vi "receiver_framev2.vi"(8 "error in (no error)":errorcluster, 9 "Timeout(100ms)":u32=100, 11 "Visa In":refnum<visa-resource-name>) -> (0 "error out":errorcluster, 1 "TimeOut?":bool, 2 "response":string, 3 "Visa out":refnum<visa-resource-name>)   [LabVIEW 2018]
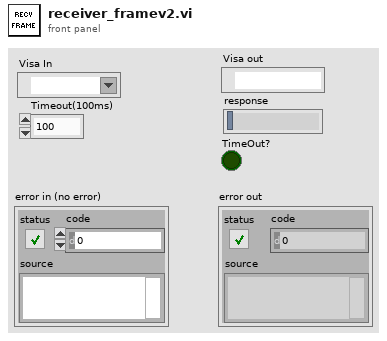
[diagram p1: front panel]
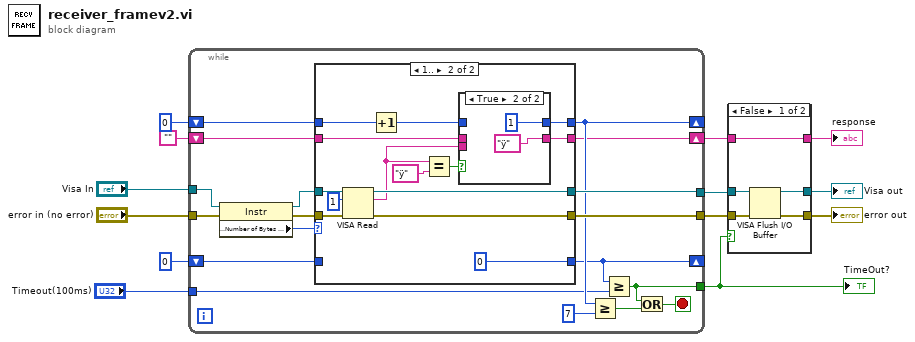
[diagram p0: block diagram]
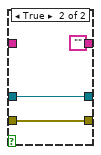
[diagram p2: hidden frame]
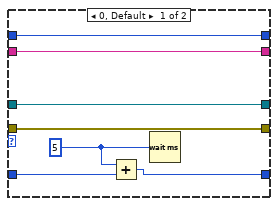
[diagram p3: hidden frame]
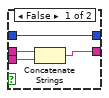
[diagram p4: hidden frame]
diagram:
  n1 = while {
    tunnel: "Visa In" -> [w31]
    tunnel: "error in (no error)" -> [w30]
    tunnel: [w26] -> w3
    tunnel: [w25] -> w7
    shift-right: [w23] -> _
    shift-left: u8 0 -> [w24]
    shift-right: [w21] -> w4
    shift-left: "" -> [w20]
    shift-right: [w14] -> _
    shift-left: u32 0 -> [w19]
    tunnel: "Timeout(100ms)" -> [w18]
    tunnel: [w15] -> w1
    stop <- w16 stop-if-true
    n2 = property class="Instr"(reference=w31, error in=w30) -> (reference out=w27:refnum<visa-resource-name>, error out=w28:errorcluster, "Serial Settings:Number of Bytes at Serial Port"=w29:u32)
    n3 = case shown="1.." w29 {
      tunnel: w28 -> [w37 w52]
      tunnel: w27 -> [w36 w51]
      tunnel: [w37 w49] -> w26
      tunnel: [w36 w48] -> w25
      tunnel: w24 -> [w38 w45]
      tunnel: [w38 w46] -> w23
      tunnel: [w35 w43] -> w21
      tunnel: w20 -> [w35 w42]
      tunnel: w19 -> [w32 _]
      tunnel: [w33 u32 0] -> w14
      frame 0, Default {
        w34 = u32 5 ("milliseconds to wait")
        n4 = Add(x=w34, y=w32) -> (x+y=w33:u32)
        n5 = Wait (ms)(milliseconds to wait=w34) -> ()  [unwired: 1 out]
      }
      frame 1.. {
        n6 = VISA Read(VISA resource name=w51, byte count=u32 1, error in (no error)=w52) -> (VISA resource name out=w48:refnum<visa-resource-name>, read buffer=w40:string, error out=w49:errorcluster)  [unwired: 1 out]
        n7 = Increment(x=w45) -> (x+1=w44:u8)
        n8 = Equal?(x=w40, y="ÿ" ("x")) -> (x = y?=w47:bool)
        n9 = case shown="True" w47 {
          tunnel: [w56 u8 1] -> w46
          tunnel: w44 -> [w56 _]
          tunnel: [w55 "ÿ" ("x")] -> w43
          tunnel: w42 -> [w54 _]
          tunnel: w40 -> [w53 _]
          frame False {
            n10 = Concatenate Strings(w54, w53) -> (w55:string)
          }
          frame True {
          }
        }
      }
    }
    n11 = Greater Or Equal?(x=w23, y=u8 7) -> (x >= y?=w17:bool)
    n12 = Greater Or Equal?(x=w14, y=w18) -> (x >= y?=w15:bool)
    n13 = Or(x=w15, y=w17) -> (x .or. y?=w16:bool)
  }
  "TimeOut?" <- w1
  n14 = case shown="False" w1 {
    tunnel: w7 -> [w63 w66]
    tunnel: [w62 w66] -> w6
    tunnel: [w61 ""] -> w5
    tunnel: w4 -> [w61 _]
    tunnel: w3 -> [w60 w64]
    tunnel: [w59 w64] -> w2
    frame False {
      n15 = VISA Flush I/O Buffer(VISA resource name=w63, error in (no error)=w60) -> (VISA resource name out=w62:refnum<visa-resource-name>, error out=w59:errorcluster)  [unwired: 1 in]
    }
    frame True {
    }
  }
  "error out" <- w2
  "Visa out" <- w6
  "response" <- w5
